vi "ZeroMQ_PUBGS.vi"() -> ()   [LabVIEW 2018]
uses:
  <vilib>/addons/zeromq/socket_type.ctl
  <vilib>/addons/zeromq/zeromq.lvlib
  <vilib>/addons/zeromq/zmq_context.lvclass
  <vilib>/addons/zeromq/zmq_socket.lvclass
panel:
  out "pub":string
  out "error out 2":errorcluster
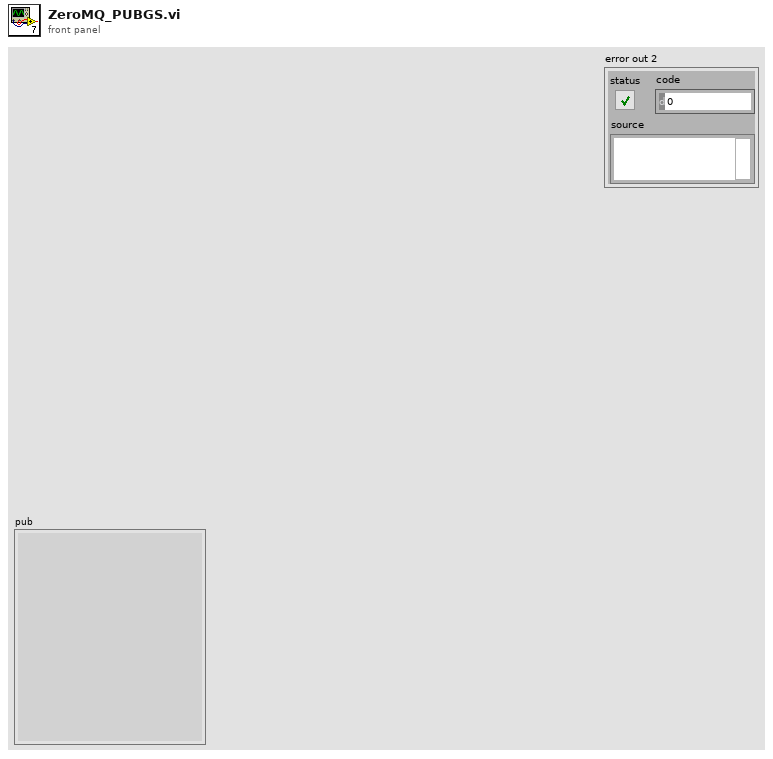
[diagram p1: front panel]
types:
  T1 = typedef "zeromq.lvlib/socket_type.ctl" = enum8{"ZMQ_PAIR", "ZMQ_PUB", "ZMQ_SUB", "ZMQ_REQ", "ZMQ_REP", "ZMQ_DEALER", "ZMQ_ROUTER", "ZMQ_PULL", "ZMQ_PUSH", "ZMQ_XPUB", "ZMQ_XSUB", "ZMQ_STREAM", "ZMQ_SERVER", "ZMQ_CLIENT", "ZMQ_RADIO", "ZMQ_DISH", "ZMQ_GATHER", "ZMQ_SCATTER", "ZMQ_DGRAM"}
  T2 = cluster{"ID":u32, "Address":string, "Service Name 1":string, "Service Name 2":string, "queue TX":refnum<queue>, "queue RX":refnum<queue>, "Port 1":u32, "Port 2":u32}
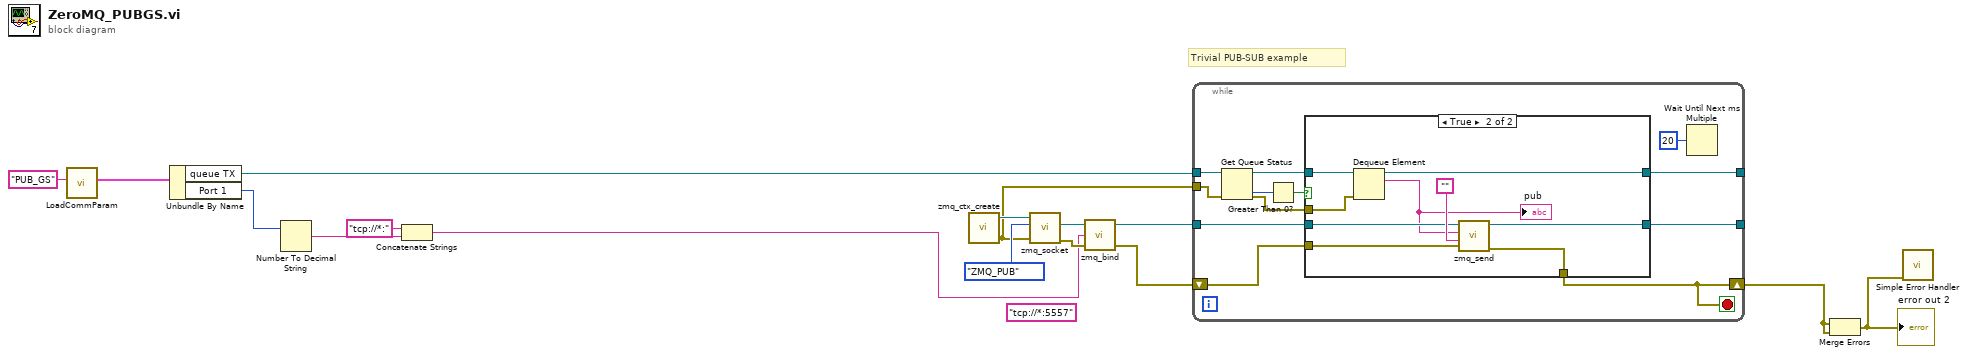
[diagram p0: block diagram]
diagram:
  (unwired) "tcp://*:5557" ("endpoint")
  # "Trivial PUB-SUB example"
  n1 = call "LoadCommParam.vi"("section name"="PUB_GS") -> ("output cluster"=w4:T2)  [unwired: 10 in]
  n2 = Unbundle By Name(w4) -> ("queue TX"=w5:refnum<queue>, "Port 1"=w9:u32)
  n3 = Number To Decimal String(number=w9) -> (decimal integer string=w8:string)  [unwired: 1 in]
  n4 = Concatenate Strings("tcp://*:" ("string"), w8) -> (w3:string)
  n5 = call <vilib>:"zmq_ctx_create.vi"() -> ("error out"=w6:errorcluster, "context out"=w16:refnum<class "zmq_context.lvclass">)  [unwired: 4 in]
  n6 = call <vilib>:"zmq_socket.vi"("error in"=w6, "socket type"=socket_type."ZMQ_PUB", "context in"=w16) -> ("error out"=w13:errorcluster, "socket out"=w14:refnum<class "zmq_socket.lvclass">)  [unwired: 2 in, 1 out]
  n7 = call <vilib>:"zmq_bind.vi"("error in"=w13, "endpoint"=w3, "socket in"=w14) -> ("error out"=w11:errorcluster, "socket out"=w12:refnum<class "zmq_socket.lvclass">)  [unwired: 1 in]
  n8 = while {
    tunnel: w12 -> [w24]
    tunnel: w5 -> [w28]
    tunnel: [w22] -> _
    tunnel: [w23] -> _
    tunnel: w6 -> [w21]
    shift-right: [w18] -> w1
    shift-left: w11 -> [w19]
    stop <- w18 stop-if-true
    n9 = Get Queue Status(queue=w28, error in (no error)=w21) -> (queue out=w27:refnum<queue>, error out=w20:errorcluster, # elements in queue=w26:i32)  [unwired: 1 in, 5 out]
    n10 = Greater Than 0?(x=w26) -> (x > 0?=w25:bool)
    n11 = case shown="True" w25 {
      tunnel: w27 -> [w30 w40]
      tunnel: w24 -> [w31 w38]
      tunnel: [w31 w36] -> w23
      tunnel: [w30 w37] -> w22
      tunnel: w20 -> [w29 w35]
      tunnel: [w29 w33] -> w18
      tunnel: w19 -> [_ w34]
      frame False {
      }
      frame True {
        n12 = Dequeue Element(queue=w40, error in (no error)=w35) -> (queue out=w37:refnum<queue>, element=w32:string)  [unwired: 1 in, 2 out]
        "pub" <- w32
        n13 = call <vilib>:"zmq_send.vi"("error in"=w34, "group"="", "data"=w32, "socket in"=w38) -> ("error out"=w33:errorcluster, "socket out"=w36:refnum<class "zmq_socket.lvclass">)  [unwired: 3 in]
      }
    }
    n14 = Wait Until Next ms Multiple(millisecond multiple=u32 20) -> ()  [unwired: 1 out]
  }
  n15 = Merge Errors(w1, w1) -> (w2:errorcluster)
  "error out 2" <- w2
  n16 = call <vilib>:"Simple Error Handler.vi"("error in (no error)"=w2) -> ()  [unwired: 4 in, 5 out]
